vi "MccHat_read.vi"(7 "n_read":i16=5, 8 "error in":errorcluster, 11 "conn_id_in":refnum<k5>) -> (0 "error out":errorcluster, 2 "readings":cluster{i32, i32, dbl}[](array[cluster]), 3 "conn_id_out":refnum<k5>, 4 "status":bool)   [LabVIEW 2019]
uses:
  <vilib>/Analysis/baseanly.llb/Mean (DBL).vi
  <vilib>/Analysis/NI_AALBase.lvlib
panel:
  out "string_raw":string
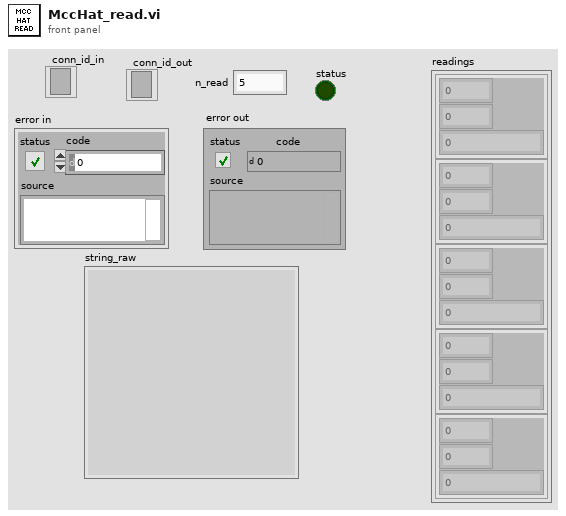
[diagram p1: front panel]
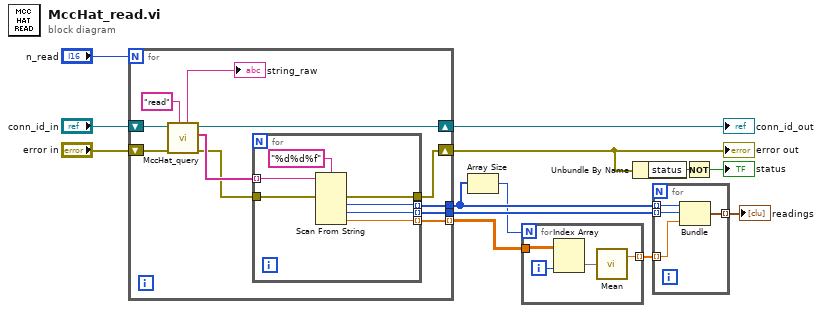
[diagram p0: block diagram]
diagram:
  n1 = for {
    N: "n_read" -> [_]
    shift-right: [w17] -> w8
    shift-left: "error in" -> [w24]
    shift-right: [w23] -> w12
    shift-left: "conn_id_in" -> [w20]
    tunnel: [w16] -> w2
    tunnel: [w15] -> w5
    tunnel: [w14] -> w6 mode=indexing
    n2 = call "MccHat_query.vi"("command"="read" ("string"), "error in"=w24, "conn_id_in"=w20) -> ("error out"=w18:errorcluster, "string_array"=w19:string[], "conn_id_out"=w23:refnum<k5>, "string_raw"=→"string_raw":string)  [unwired: 4 in, 1 out]
    n3 = for {
      tunnel: w19 -> [w31] mode=indexing
      tunnel: w18 -> [w29]
      tunnel: [w28] -> w17
      tunnel: [w27] -> w16 mode=indexing
      tunnel: [w26] -> w15 mode=indexing
      tunnel: [w25] -> w14 mode=indexing
      n4 = Scan From String(format string="%d%d%f", input string=w31, error in=w29) -> (error out=w28:errorcluster, output 1=w27:i32, output 2=w26:i32, output 3=w25:dbl)  [unwired: 4 in, 2 out]
    }
  }
  "error out" <- w8
  "conn_id_out" <- w12
  n5 = Array Size(array=w2) -> (size(s)=w1:i32)
  n6 = for {
    N: w1 -> [_]
    tunnel: w6 -> [w35]
    tunnel: [w32] -> w4 mode=indexing
    i -> [w34]
    n7 = Index Array(array=w35, index (col)=w34) -> (element=w33:dbl[])  [unwired: 1 in]
    n8 = call-poly <vilib>:"Mean.vi"("X"=w33) -> ("mean"=w32:dbl)  [unwired: 1 out]
  }
  n9 = Unbundle By Name(w8) -> ("status"=w10:bool)
  n10 = for {
    tunnel: w2 -> [w39] mode=indexing
    tunnel: w5 -> [w38] mode=indexing
    tunnel: w4 -> [w37] mode=indexing
    tunnel: [w36] -> w3 mode=indexing
    n11 = Bundle(w39, w38, "mean"=w37) -> (w36:cluster{i32, i32, "mean":dbl})  [unwired: 1 in]
  }
  "readings" <- w3
  n12 = Not(x=w10) -> (.not. x?=→"status":bool)
